vi "Configure Voltage.vi"(8 "error in (no error)":errorcluster, 10 "Voltage":dbl, 11 "Manual PSU in":refnum<class "Manual PSU.lvclass">) -> (0 "error out":errorcluster, 3 "Manual PSU out":refnum<class "Manual PSU.lvclass">)   [LabVIEW 2020, in "Manual PSU.lvclass"]
uses:
  Manual PSU.lvclass
  C:/Sandbox/RF Bench/Source Code/WiSpry Test Framework/Instruments/Power Supply/Power Supply.lvclass
  Power Supply.lvclass/Power Supply.ctl
  Power Supply.lvclass
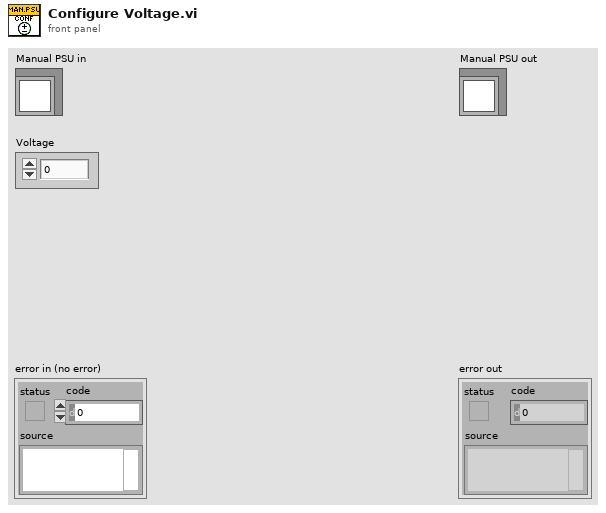
[diagram p1: front panel]
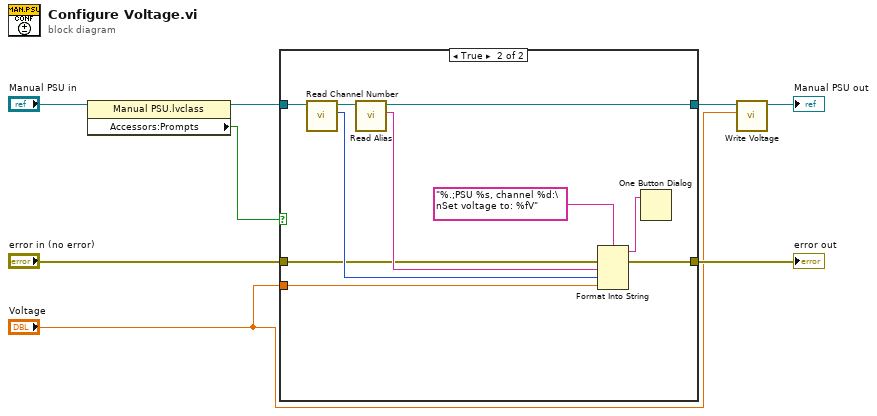
[diagram p0: block diagram]
diagram:
  n1 = property class="Manual PSU.lvclass"(reference="Manual PSU in") -> (reference out=w4:refnum<class "Manual PSU.lvclass">, "Accessors:Prompts"=w6:bool)  [unwired: 1 in, 1 out]
  n2 = case shown="True" w6 {
    tunnel: w4 -> [w10 w15]
    tunnel: [w10 w14] -> w3
    tunnel: [w9 w13] -> w8
    tunnel: "error in (no error)" -> [w9 w12]
    tunnel: "Voltage" -> [_ w11]
    frame False {
    }
    frame True {
      n3 = call "Read Channel Number.vi"("Power Supply in"=w15) -> ("Channel Number"=w16:u8, "Power Supply out"=w17:refnum<class "Manual PSU.lvclass">)  [unwired: 9 in]
      n4 = call-dynamic "Read Alias.vi"("Power Supply in"=w17) -> ("Alias"=w18:string, "Power Supply out"=w14:refnum<class "Manual PSU.lvclass">)  [unwired: 9 in]
      n5 = Format Into String(format string="%.;PSU %s, channel %d:\nSet voltage to: %fV", error in=w12, w18, w16, w11) -> (resulting string=w19:string, error out=w13:errorcluster)  [unwired: 1 in]
      n6 = One Button Dialog(message=w19) -> ()  [unwired: 1 in, 1 out]
    }
  }
  "error out" <- w8
  n7 = call "Write Voltage.vi"("Voltage"="Voltage", "Power Supply in"=w3) -> ("Power Supply out"=→"Manual PSU out":refnum<class "Manual PSU.lvclass">)  [unwired: 9 in]
